vi "Get Scanner.vi"(8 "error in (no error)":errorcluster, 11 "Scannable in":refnum<class "Scannable.lvclass">) -> (0 "error out":errorcluster, 2 "Default Scanner out":refnum<class "Scanner.lvclass">)   [LabVIEW 2012, in "Scannable.lvclass"]
doc: "(Dynamic) Returns the default Scanner object that scans over this Scannable. (Note that a Scannable may have multiple Scanners associated with it.) A Scanner is an analogue to an Iterator class in other languages."
uses:
  Scannable.lvclass
  Scanners/Scanner/Scanner.lvclass
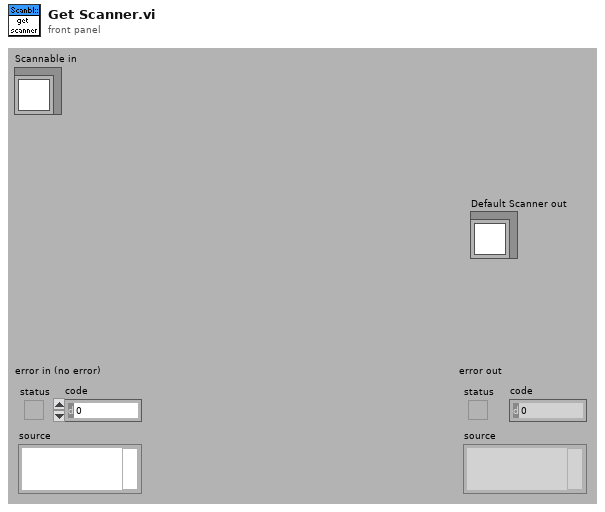
[diagram p1: front panel]
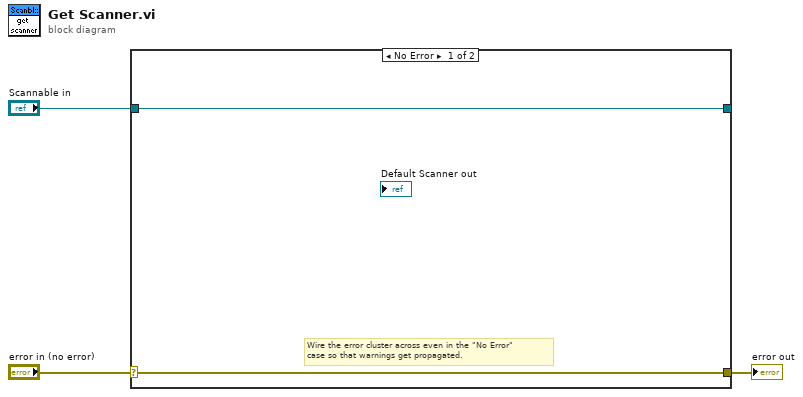
[diagram p0: block diagram]
diagram:
  n1 = case shown="No Error" "error in (no error)" {
    selector: "error in (no error)" -> [w4 w7]
    tunnel: [w4 w7] -> w2
    tunnel: [w5 w6] -> _
    tunnel: "Scannable in" -> [w5 w6]
    frame No Error {
      # "Wire the error cluster across even in the \"No Error\"\ncase so that warnings get propagated."
    }
    frame Error {
    }
  }
  "error out" <- w2
